vi "Add enum Type to JSON Schema.vi"(8 "error in (no error)":errorcluster, 11 "JSON Schema in":string) -> (0 "error out":errorcluster, 3 "JSON Schema out":string)   [LabVIEW 2019, in "JSON-Schema.lvlib"]
uses:
  JSON-Schema.lvlib
  <vilib>/JDP Science/JSONtext/Next JSON Value.vi
  <vilib>/JDP Science/JSONtext/String Subset.vi
  <vilib>/JDP Science/JSONtext/Parsing/Advance past next JSON Value (inlined COPY).vi
  <vilib>/JDP Science/JSONtext/Parsing/Advance past whitespace.vi
  <vilib>/JDP Science/JSONtext/Parsing/Advance past String.vi
  <vilib>/JDP Science/JSONtext/Parsing/Advance past Number.vi
  <vilib>/JDP Science/JSONtext/Parsing/Advance past Line Ending.vi
  <vilib>/JDP Science/JSONtext/Parsing/Parse Full Path or Item Name.vi
  <vilib>/JDP Science/JSONtext/Parsing/Advance past Array.vi
  <vilib>/JDP Science/JSONtext/Parsing/Advance past Object.vi
  <vilib>/JDP Science/JSONtext/support/Error Cluster From Code.vi
  <vilib>/JDP Science/JSONtext/Offset/Find Item Locations by Path.vi
  <vilib>/JDP Science/JSONtext/JSONtext.lvlib
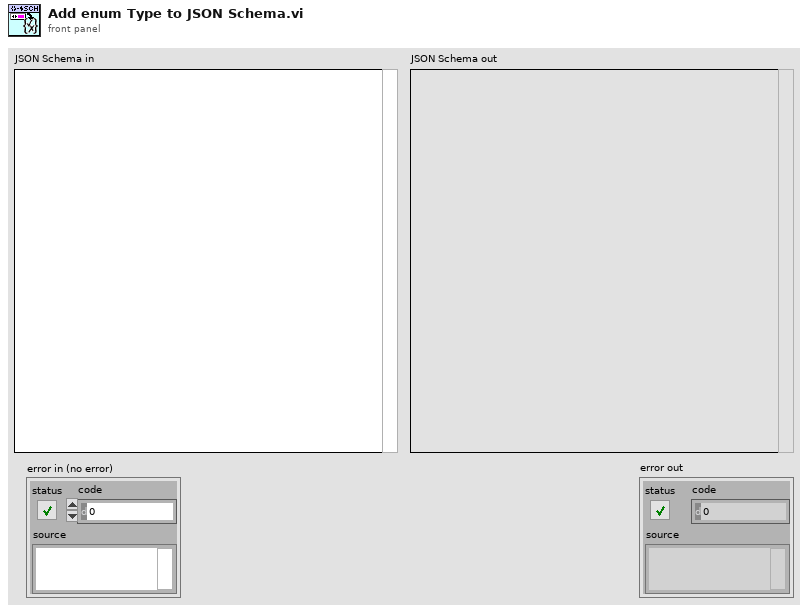
[diagram p1: front panel]
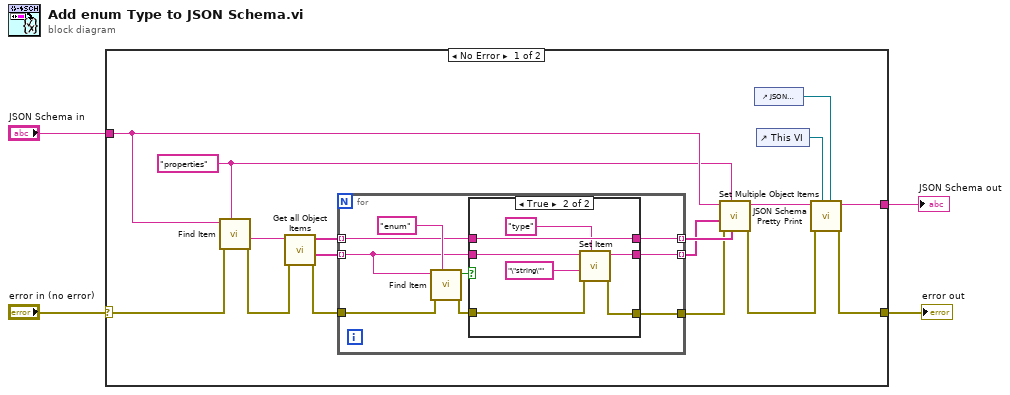
[diagram p0: block diagram]
diagram:
  n1 = case shown="No Error" "error in (no error)" {
    selector: "error in (no error)" -> [w12 w41]
    tunnel: "JSON Schema in" -> [w19 _]
    tunnel: [w7 w41] -> w2
    tunnel: [w8 _] -> w1
    frame No Error {
      w18 = "properties" ("$Path or Item Name")
      n2 = call <vilib>:"Find Item.vi"("$Path or Item Name"=w18, "error in (no error)"=w12, "JSON"=w19) -> ("error out"=w14:errorcluster, "<JSON>"=w13:string)  [unwired: 5 in, 2 out]
      n3 = call <vilib>:"Get all Object Items.vi"("error in (no error)"=w14, "JSON"=w13) -> ("error out"=w17:errorcluster, "<JSON>"=w15:string[], "Item Names"=w16:string[])  [unwired: 6 in, 1 out]
      n4 = for {
        tunnel: w15 -> [w28] mode=indexing
        tunnel: w16 -> [w27] mode=indexing
        tunnel: w17 -> [w29]
        tunnel: [w24] -> w20 mode=indexing
        tunnel: [w23] -> w21 mode=indexing
        tunnel: [w22] -> w11
        n5 = call <vilib>:"Find Item.vi"("$Path or Item Name"="enum", "error in (no error)"=w29, "JSON"=w28) -> ("error out"=w25:errorcluster, "Found"=w26:bool)  [unwired: 5 in, 2 out]
        n6 = case shown="True" w26 {
          tunnel: w28 -> [w33 w39]
          tunnel: w27 -> [w32 w36]
          tunnel: w25 -> [w31 w38]
          tunnel: [w33 w37] -> w24
          tunnel: [w32 w36] -> w23
          tunnel: [w31 w34] -> w22
          frame False {
          }
          frame True {
            n7 = call <vilib>:"Set Item.vi"("$Path or Item Name"="type", "error in (no error)"=w38, "JSON to Insert"="\"string\"" ("$Path or Item Name"), "JSON"=w39) -> ("error out"=w34:errorcluster, "<JSON>"=w37:string)  [unwired: 4 in, 1 out]
          }
        }
      }
      n8 = call <vilib>:"Set Multiple Object Items.vi"("Item Names"=w21, "$Path or Item Name"=w18, "error in (no error)"=w11, "JSON Items"=w20, "JSON"=w19) -> ("error out"=w9:errorcluster, "<JSON>"=w10:string)  [unwired: 4 in]
      n9 = control-ref of="JSON Schema out"() -> (w5:refnum<vi>)
      n10 = control-ref of="This VI"() -> (w6:refnum<vi>)
      n11 = call "JSON Schema Pretty Print.vi"("String Control"=w5, "reference"=w6, "error in (no error)"=w9, "<JSON> in"=w10) -> ("error out"=w7:errorcluster, "<JSON> out"=w8:string)  [unwired: 6 in]
    }
    frame Error {
    }
  }
  "JSON Schema out" <- w1
  "error out" <- w2
